vi "Get Program Errors.vi"(8 "Error In":errorcluster, 10 "Program Handle":T1, 11 "Device In":T2) -> (0 "Error Out":errorcluster, 1 "Compile Log":string, 2 "Program Out":T1, 3 "Device Out":T2)   [LabVIEW 2012, in "OpenCLV x64.lvlib"]
doc: "Gets the OpenCL compiler errors produced by a program."
uses:
  OpenCLV x64.lvlib
  Controls/Device ID.ctl
  Controls/Program Handle.ctl
  Error Checking/Add Error Functional Global.vi
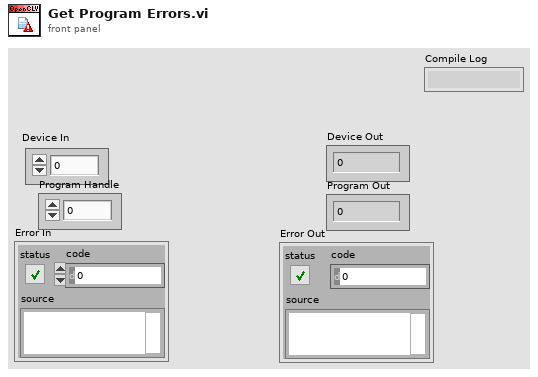
[diagram p1: front panel]
types:
  T1 = typedef "OpenCLV x64.lvlib/Program Handle.ctl" = u64
  T2 = typedef "OpenCLV x64.lvlib/Device ID.ctl" = u64
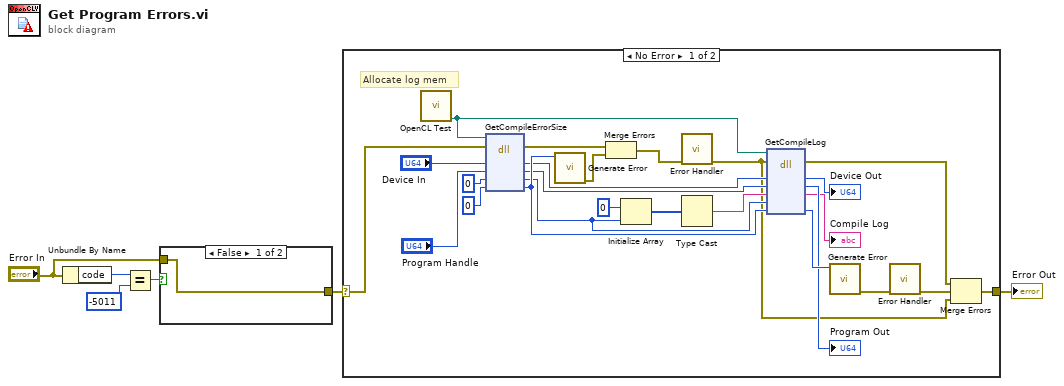
[diagram p0: block diagram]
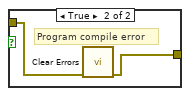
[diagram p2: hidden frame]
diagram:
  n1 = Unbundle By Name("Error In") -> ("code"=w5:i32)
  n2 = Equal?(x=w5, y=-5011) -> (x = y?=w3:bool)
  n3 = case shown="False" w3 {
    tunnel: "Error In" -> [w7 w9]
    tunnel: [w7 w8] -> w1
    frame False {
    }
    frame True {
      # "Program compile error"
      n4 = call <vilib>:"Clear Errors.vi"("error in (no error)"=w9) -> ("error out"=w8:errorcluster)  [unwired: 6 in]
    }
  }
  n5 = case shown="No Error" w1 {
    selector: w1 -> [w10 w35]
    tunnel: [w19 w35] -> w6
    frame No Error {
      # "Allocate log mem"
      n6 = call "OpenCL Test.vi"() -> ("DLL To Use"=w18:path)  [unwired: 11 in]
      n7 = dll-call lib="C:/Users/bme-amcelroy-la/Desktop/OpenCLV/trunk/OpenCLV_x64_1.0/OpenCLV_x64.dll" fn="GetCompileErrorSize"(path in=w18, error in=w10, "Device In"="Device In", "Program Handle"="Program Handle", "Log Size"=u64 0, "Error"=0) -> (error out=w11:errorcluster, "Device In"=w27:u64, "Program Handle"=w28:u64, "Log Size"=w32:u64, "Error"=w34:i32)  [unwired: 2 in, 1 out]
      n8 = call "Generate Error.vi"("Error"=w34) -> ("error out"=w13:errorcluster)  [unwired: 10 in]
      n9 = Merge Errors(w11, w13) -> (w12:errorcluster)
      n10 = Initialize Array(u8 0 ("Error"), w32) -> (w30:u8[])
      n11 = call-poly "Error Handler.vi"("Error In"=w12) -> ("Error Out"=w17:errorcluster)  [unwired: 10 in]
      n12 = Type Cast(x=w30) -> (*(type *) &x=w31:string)  [unwired: 1 in]
      n13 = dll-call lib="D:/OpenCLV/trunk/OpenCLV_x64_1.0/OpenCLV_x64.dll" fn="GetCompileLog"(path in=w18, error in=w17, "Device In"=w27, "Program Handle"=w28, "Compile Log"=w31, "Log Size"=w32, "Error"=w34) -> (error out=w14:errorcluster, "Device In"=→"Device Out":u64, "Program Handle"=→"Program Out":u64, "Compile Log"=→"Compile Log":string, "Error"=w33:i32)  [unwired: 3 in, 1 out]
      n14 = call "Generate Error.vi"("Error"=w33) -> ("error out"=w16:errorcluster)  [unwired: 10 in]
      n15 = call-poly "Error Handler.vi"("Error In"=w16) -> ("Error Out"=w15:errorcluster)  [unwired: 10 in]
      n16 = Merge Errors(w14, w15, w17) -> (w19:errorcluster)
    }
    frame Error {
    }
  }
  "Error Out" <- w6
